vi "Auton Warmup Shooter.vi"(11 "Shot Type":i32) -> ()   [LabVIEW 2015]
uses:
  Robot Global Data.vi
  Common Code/Shoot Modes Enum.ctl
  Common Code/Catapult/Catapult Auto Commands.ctl
  Common Code/Shot Type.ctl
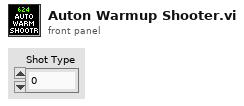
[diagram p1: front panel]
types:
  T1 = typedef "Shooter Commands.ctl" = enum16{"Idle", "Prime Shooter", "Shoot"}
  T2 = typedef "Shoot Modes Enum.ctl" = enum16{"Manual", "Auto"}
  T3 = typedef "Shot Type.ctl" = enum16{"Batter Shot", "Corner Shot", "Cleat Shot", "Vision Shot", "Deep Middle Shot"}
  T4 = typedef "Shooter Command Cluster.ctl" = cluster{"Command":T5, "Mode":T2, "Shot Type":T3, "Override Trigger Sensor":bool, "Override Angle?":bool, "Hide From Death":bool}
  T5 = typedef "Catapult Auto Commands.ctl" = enum16{"Idle", "Warmup", "Shoot"}
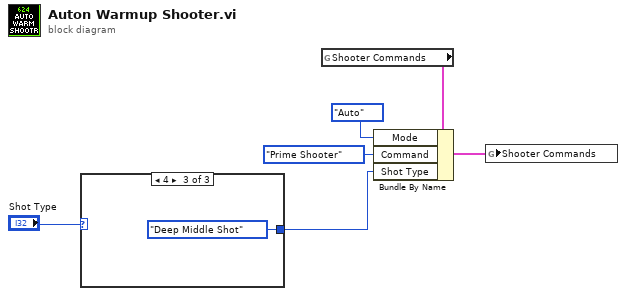
[diagram p0: block diagram]
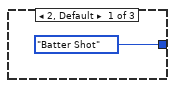
[diagram p2: hidden frame]
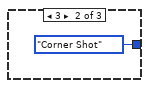
[diagram p3: hidden frame]
diagram:
  n1 = case shown="4" "Shot Type" {
    tunnel: [Shot_Type."Batter Shot" ("Shot Type") Shot_Type."Corner Shot" ("Shot Type") Shot_Type."Deep Middle Shot" ("Shot Type")] -> w1
    frame 2, Default {
    }
    frame 3 {
    }
    frame 4 {
    }
  }
  n2 = global read "Robot Global Data.vi" "Shooter Commands"() -> (w5:T4)
  n3 = Bundle By Name(cluster=w5, "Mode"=Shoot_Modes_Enum."Auto", "Command"=Shooter_Commands."Prime Shooter", "Shot Type"=w1) -> (w6:T4)
  n4 = global write "Robot Global Data.vi" "Shooter Commands"(w6) -> ()
